vi "Ex_Write.vi"() -> ()   [LabVIEW 2015]
doc: "X-CAN example VI that continually writes data to the X-CAN device using an X-CAN Session. Every write iteration the X-CAN LEDs will be toggled."
uses:
  <vilib>/Stratom, Inc/X-CAN for myRIO (API)/X-CAN Class/Type Definitions/CANFrame.ctl
  <vilib>/Stratom, Inc/X-Modules for myRIO/Type Defs/MXPChannel.ctl
  <vilib>/Stratom, Inc/X-CAN for myRIO (API)/X-CAN Class/Type Definitions/CAN_Speed.ctl
  <vilib>/Platform/TimedLoop/XDataNode/timing_clust.ctl
  <vilib>/Platform/TimedLoop/XDataNode/nitl_modes.ctl
  <vilib>/Platform/TimedLoop/XDataNode/wakeup.ctl
  Control/State_Write.ctl
  <vilib>/Stratom, Inc/X-CAN for myRIO (API)/X-CAN Class/X-CAN.lvclass
  <vilib>/Platform/TimedLoop/XDataNode/XDataNode.xnode
  <vilib>/Platform/TimedLoop/XDataNode/XDNodeRunTimeDep.lvlib
panel:
  in  "OK Button":bool
  in  "CAN Frame":T1={"identifier"=0, "extended?"=FALSE, "echo?"=FALSE, "payload"=[0, 0, 0, 0, 0, 0, 0, 0], "timestamp"=timestamp(0 s since 1904-01-01)} {"payload" format="%x"; "timestamp" format="%<%I:%M:%S%8u %p\n%x>T"; "identifier" format="%x"}
  in  "Stop Button":bool
  # "X-CAN Write"
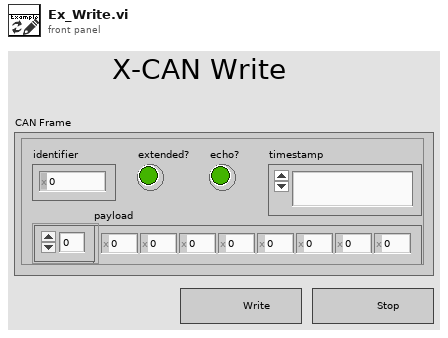
[diagram p1: front panel]
types:
  T1 = typedef "X-CAN.lvclass/CANFrame.ctl" = cluster{"identifier":u32, "extended?":bool, "echo?":bool, "payload":u8[], "timestamp":timestamp}
  T2 = typedef "State_Write.ctl" = enum16{"Idle", "Write", "Stop"}
  T3 = typedef "X-CAN.lvclass/CAN_Speed.ctl" = u8
  T4 = typedef "MXPChannel.ctl" = enum16{"A/MXP", "B/MXP"}
  T5 = typedef "XDNodeRunTimeDep.lvlib/timing_clust.ctl" = cluster{"Expected End [f-1]":u64, "Actual End [f-1]":u64, "Finished Late? [f-1]":bool, "Expected End [i-1]":u64, "Actual End [i-1]":u64, "Finished Late? [i-1]":bool, "Expected Start [i]":u64, "Actual Start [i]":u64, "Expected Start [f]":u64, "Actual Start [f]":u64, "Source Name":string, "Structure Name":string, "Period":i64, "Deadline":i64, "Offset":i64, "Start":i64, "Priority":i32, "Timeout":i32, "Mode":T6, "Wakeup Reason":T7, "Error":errorcluster, "Source Type":string, "Secondary Source Type":string, "Global End Time":u64, "Global Start Time":u64, "Frame Duration":u64, "Iteration Duration":u64, "Assigned CPU":i32, "I/O Scan Engine Mode":u32}
  T6 = typedef "XDNodeRunTimeDep.lvlib/nitl_modes.ctl" = enum32{"No Change", "Process missed periods, maintain original phase", "Discard missed periods, maintain original phase", "Process missed periods, ignore original phase", "Discard missed periods, ignore original phase"}
  T7 = typedef "XDNodeRunTimeDep.lvlib/wakeup.ctl" = enum32{"Normal", "Aborted", "Asynchronous wakeup", "Timing source error", "Timed loop error", "Timeout"}
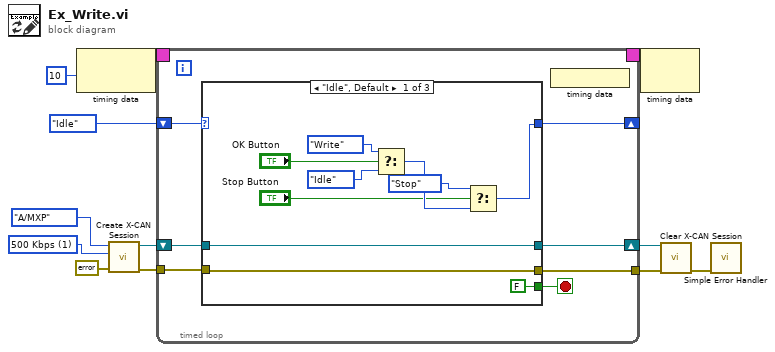
[diagram p0: block diagram]
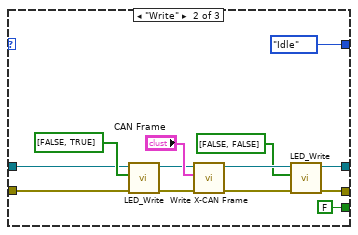
[diagram p2: hidden frame]
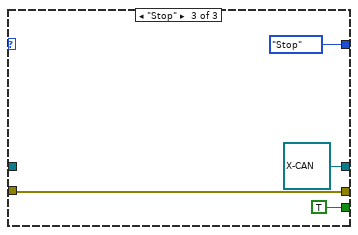
[diagram p3: hidden frame]
diagram:
  w7 = T3 1 items=["125 Kbps"=7, "250 Kbps"=3, "500 Kbps"=1, "1000 Kbps"=0, "95.238 Kbps"=6] ("CAN Speed [Kbps]")
  n1 = node-c288(i64 10 ("Period")) -> (w12:T5)
  n2 = call <vilib>:"Create X-CAN Session.vi"("error in (no error)"=errorcluster {"status"=FALSE, "code"=0, "source"=""}, "CAN Speed [Kbps]"=w7, "MXP Channel"=MXPChannel."A/MXP") -> ("error out"=w10:errorcluster, "X-CAN Session out"=w3:refnum<class "X-CAN.lvclass">)  [unwired: 7 in]
  n3 = timed-loop {
    timing: w12 -> [_]
    timing-out: [_] -> w11
    tunnel: w10 -> [w18]
    shift-right: [w15] -> w5
    shift-left: w3 -> [w17]
    tunnel: [w19] -> w6
    shift-right: [w14] -> _
    shift-left: State_Write."Idle" -> [w16]
    stop <- w13 stop-if-true
    n4 = case shown="\"Idle\", Default" w16 {
      tunnel: [w21 w37 w44] -> w19
      tunnel: w18 -> [w21 w40 w44]
      tunnel: w17 -> [w22 w33 _]
      tunnel: [w22 w36 refnum<class "X-CAN.lvclass"> refnum ("X-CAN out")] -> w15
      tunnel: [w23 State_Write."Idle" State_Write."Stop"] -> w14
      tunnel: [FALSE FALSE TRUE] -> w13
      frame "Idle", Default {
        n5 = Select(t=State_Write."Write", s="OK Button", f=State_Write."Idle") -> (s? t:f=w26:T2)
        n6 = Select(t=State_Write."Stop", s="Stop Button", f=w26) -> (s? t:f=w23:T2)
      }
      frame "Write" {
        n7 = call <vilib>:"LED_Write.vi"("error in"=w40, "LED Values"=bool[] [FALSE, TRUE], "X-CAN in"=w33) -> ("error out"=w39:errorcluster, "X-CAN out"=w34:refnum<class "X-CAN.lvclass">)  [unwired: 7 in]
        n8 = call <vilib>:"Write X-CAN Frame.vi"("error in"=w39, "CAN Frame"="CAN Frame", "X-CAN Session in"=w34) -> ("error out"=w38:errorcluster, "X-CAN Session out"=w35:refnum<class "X-CAN.lvclass">)  [unwired: 7 in]
        n9 = call <vilib>:"LED_Write.vi"("error in"=w38, "LED Values"=bool[] [FALSE, FALSE], "X-CAN in"=w35) -> ("error out"=w37:errorcluster, "X-CAN out"=w36:refnum<class "X-CAN.lvclass">)  [unwired: 7 in]
      }
      frame "Stop" {
      }
    }
    n10 = node-c288() -> ()  [unwired: 1 out]
  }
  n11 = node-c288(w11) -> ()  [unwired: 1 out]
  n12 = call <vilib>:"Clear X-CAN Session.vi"("error in (no error)"=w6, "X-CAN Session in"=w5) -> ("error out"=w4:errorcluster)  [unwired: 9 in]
  n13 = call <vilib>:"Simple Error Handler.vi"("error in (no error)"=w4) -> ()  [unwired: 4 in, 5 out]
